vi "datetimearray_to_reltime.vi"(10 "Date Array":string[](array[string]), 11 "Time Array":string[](array[string])) -> (3 "Rel. time array":dbl[](array[numeric]))   [LabVIEW 2022 SP3]
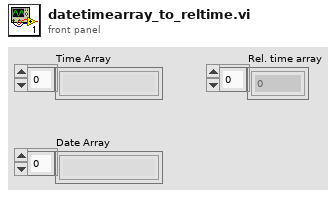
[diagram p1: front panel]
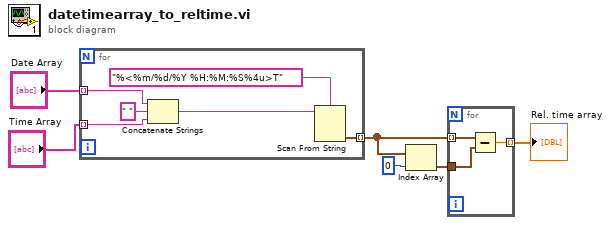
[diagram p0: block diagram]
diagram:
  n1 = for {
    tunnel: "Time Array" -> [w7] mode=indexing
    tunnel: "Date Array" -> [w8] mode=indexing
    tunnel: [w9] -> w5 mode=indexing
    n2 = Concatenate Strings(w8, " " ("string"), w7) -> (w11:string)
    n3 = Scan From String(format string="%<%m/%d/%Y %H:%M:%S%4u>T" ("time format string (%c)"), input string=w11) -> (output 1=w9:timestamp)  [unwired: 3 in, 3 out]
  }
  n4 = Index Array(array=w5, index=0 ("disabled index (col)")) -> (element=w4:timestamp)
  n5 = for {
    tunnel: w5 -> [w14] mode=indexing
    tunnel: w4 -> [w15]
    tunnel: [w13] -> w6 mode=indexing
    n6 = Subtract(x=w14, y=w15) -> (x-y=w13:dbl)
  }
  "Rel. time array" <- w6
